vi "create initial guess assuming vertical magnet.vi"(7 "board inverted?":bool, 10 "Br*V (T*mm^3)":dbl=500.0, 11 "Magnetometer reading set":T1) -> (3 "initial guess":T2)   [LabVIEW 2017]
uses:
  typedefs/magnet location fit result.ctl
  typedefs/magnetomter reading set.ctl
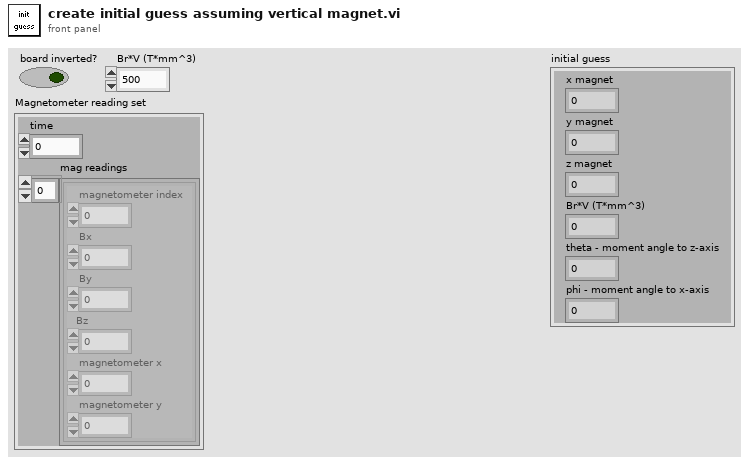
[diagram p1: front panel]
types:
  T1 = typedef "magnetomter reading set.ctl" = cluster{"time":fxp<+,48,48>, "mag readings":cluster{"magnetometer index":dbl, "Bx":dbl, "By":dbl, "Bz":dbl, "magnetometer x":dbl, "magnetometer y":dbl}[]}
  T2 = typedef "magnet location fit result.ctl" = cluster{"x magnet":dbl, "y magnet":dbl, "z magnet":dbl, "Br*V (T*mm^3)":dbl, "theta - moment angle to z-axis":dbl, "phi - moment angle to x-axis":dbl}
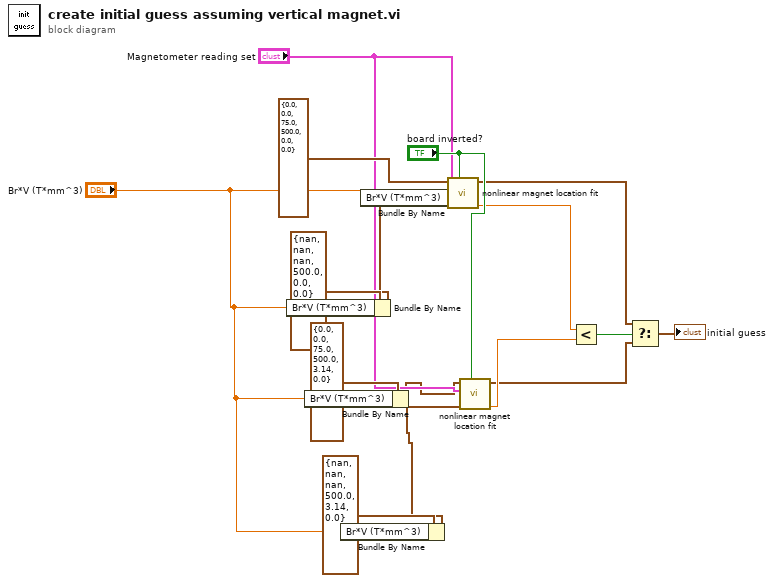
[diagram p0: block diagram]
diagram:
  n1 = Bundle By Name(cluster=T2 {"x magnet"=nan, "y magnet"=nan, "z magnet"=nan, "Br*V (T*mm^3)"=500.0, "theta - moment angle to z-axis"=0.0, "phi - moment angle to x-axis"=0.0} ("fixed parameters"), "Br*V (T*mm^3)"="Br*V (T*mm^3)") -> (w4:T2)
  n2 = Bundle By Name(cluster=T2 {"x magnet"=0.0, "y magnet"=0.0, "z magnet"=75.0, "Br*V (T*mm^3)"=500.0, "theta - moment angle to z-axis"=3.14, "phi - moment angle to x-axis"=0.0} ("initial parameters"), "Br*V (T*mm^3)"="Br*V (T*mm^3)") -> (w3:T2)
  n3 = Bundle By Name(cluster=T2 {"x magnet"=nan, "y magnet"=nan, "z magnet"=nan, "Br*V (T*mm^3)"=500.0, "theta - moment angle to z-axis"=3.14, "phi - moment angle to x-axis"=0.0} ("fixed parameters"), "Br*V (T*mm^3)"="Br*V (T*mm^3)") -> (w2:T2)
  n4 = Bundle By Name(cluster=T2 {"x magnet"=0.0, "y magnet"=0.0, "z magnet"=75.0, "Br*V (T*mm^3)"=500.0, "theta - moment angle to z-axis"=0.0, "phi - moment angle to x-axis"=0.0} ("initial parameters"), "Br*V (T*mm^3)"="Br*V (T*mm^3)") -> (w5:T2)
  n5 = call "nonlinear magnet location fit.vi"("board inverted?"="board inverted?", "fixed parameters"=w4, "Magnetometer reading set"="Magnetometer reading set", "initial parameters"=w5) -> ("residue"=w11:dbl, "fit parameters"=w9:T2)  [unwired: 5 in, 1 out]
  n6 = call "nonlinear magnet location fit.vi"("board inverted?"="board inverted?", "fixed parameters"=w2, "Magnetometer reading set"="Magnetometer reading set", "initial parameters"=w3) -> ("residue"=w12:dbl, "fit parameters"=w8:T2)  [unwired: 5 in, 1 out]
  n7 = Less?(x=w11, y=w12) -> (x < y?=w10:bool)
  n8 = Select(t=w9, s=w10, f=w8) -> (s? t:f=→"initial guess":T2)
